vi "Global Mapper F.vi"(8 "picture in":picture, 11 "GIC Input":T1={"     Use ?\nOff       On"=[FALSE, TRUE, FALSE, TRUE], "Mode:"=FALSE, "WP Data"="", "Hokuyo Port"="COM7", "Prop  Port"="COM6", "Compass Port"="", "GPS Port"="", "Num of WPs"=0, "WP Lats and Longs"={"WP Lats"=[], "WP Longs"=[]}, "Obst Lats and Longs"={"Obst Lats"=[], "Obst Longs"=[]}, "Parameters"=[], "GPS Data"=[], "Compass"=0.0, "LMS Vector"=[], "Vision Vector"=[], "Direction Cmd"=0.0, "Speed Cmd"=0.0, "WP Vector"=[], "WP Number"=0, "Extra"=0, "SW Map"=[], "Path Cluster"={"Path x node"=[], "Path y node"=[]}, "Sim Course"=[]} {"Obst Lats and Longs"."Obst Longs" format="%#_8g"; "Obst Lats and Longs"."Obst Lats" format="%#_8g"}) -> (0 "picture out":picture)   [LabVIEW 2014]
panel:
  # "Global Mapper F"
  # "Inputs:"
  # "Output:"
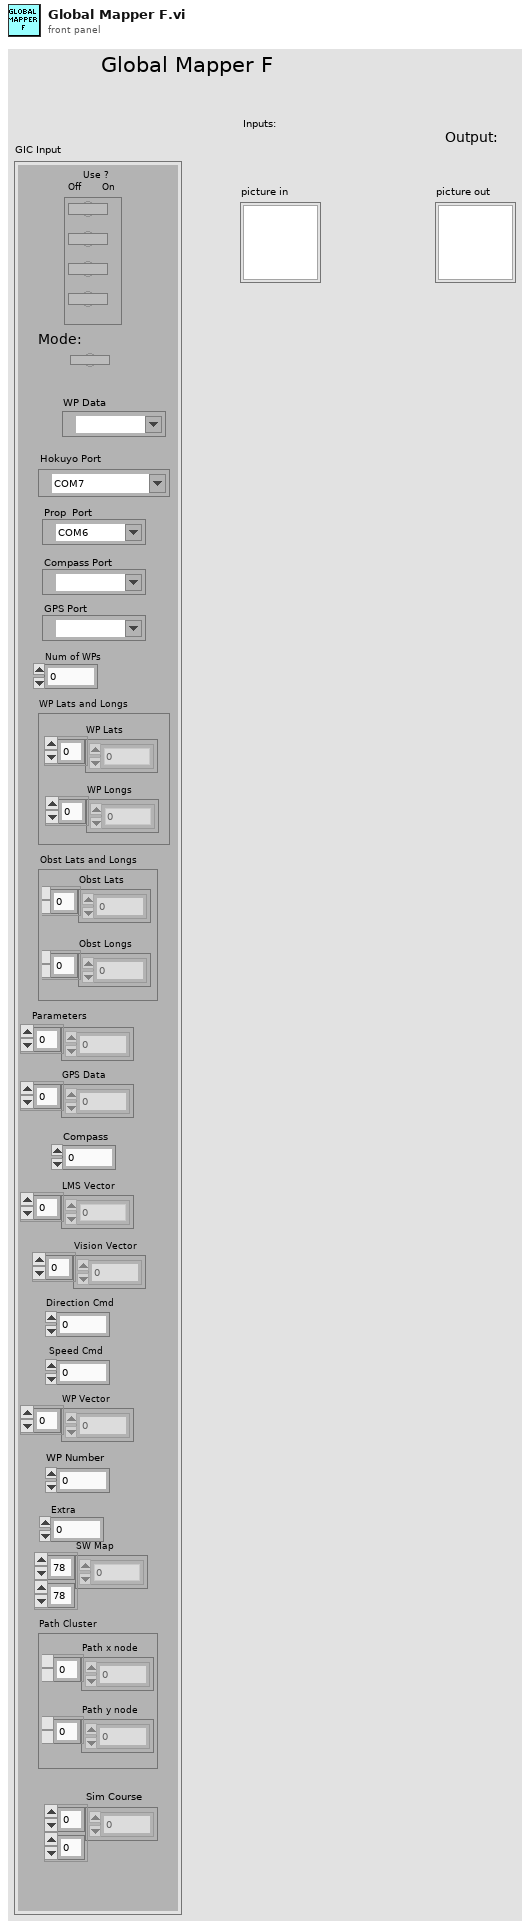
[diagram p1: front panel]
types:
  T1 = cluster{"     Use ?\nOff       On":bool[], "Mode:":bool, "WP Data":refnum<visa-resource-name>, "Hokuyo Port":refnum<visa-resource-name>, "Prop  Port":refnum<visa-resource-name>, "Compass Port":refnum<visa-resource-name>, "GPS Port":refnum<visa-resource-name>, "Num of WPs":i16, "WP Lats and Longs":cluster{"WP Lats":dbl[], "WP Longs":dbl[]}, "Obst Lats and Longs":cluster{"Obst Lats":dbl[], "Obst Longs":dbl[]}, "Parameters":dbl[], "GPS Data":dbl[], "Compass":dbl, "LMS Vector":dbl[], "Vision Vector":dbl[], "Direction Cmd":dbl, "Speed Cmd":dbl, "WP Vector":dbl[], "WP Number":i32, "Extra":i16, "SW Map":i32[][], "Path Cluster":cluster{"Path x node":dbl[], "Path y node":dbl[]}, "Sim Course":i8[][]}
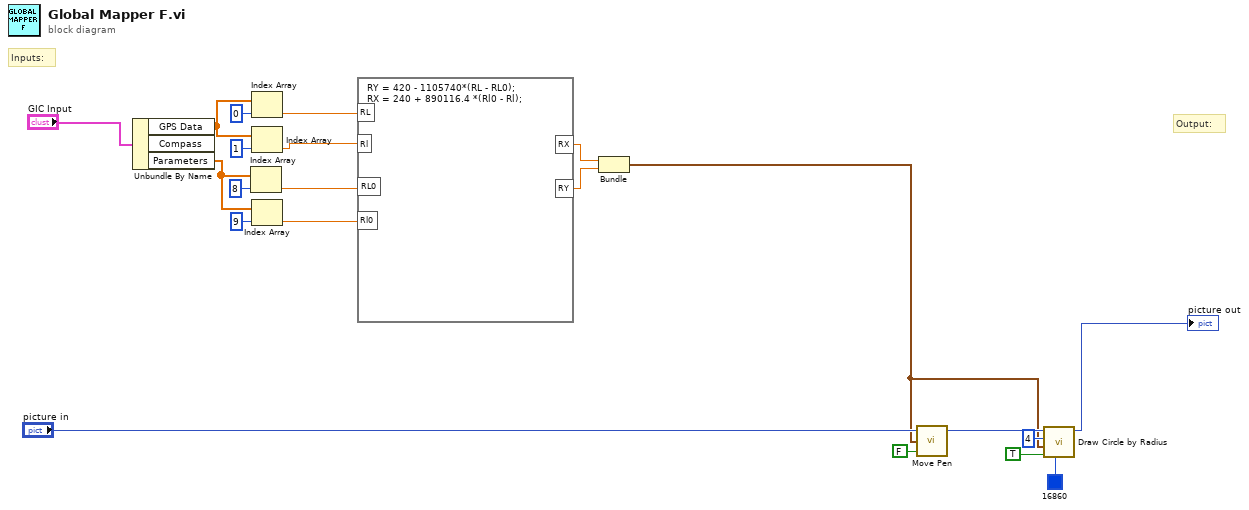
[diagram p0: block diagram]
diagram:
  # "Output:"
  # "Inputs:"
  n1 = Unbundle By Name("GIC Input") -> ("GPS Data"=w18:dbl[], "Parameters"=w13:dbl[])  [unwired: 1 out]
  n2 = Index Array(array=w13, index=8) -> (element=w15:dbl)
  n3 = Index Array(array=w18, index=0) -> (element=w20:dbl)
  n4 = Index Array(array=w18, index=1) -> (element=w16:dbl)
  n5 = Index Array(array=w13, index=9) -> (element=w11:dbl)
  n6 = formula code="RY = 420 - 1105740*(RL - RL0);\nRX = 240 + 890116.4 *(Rl0 - Rl);"("RL"=w20, "Rl"=w16, "RL0"=w15, "Rl0"=w11) -> ("RY"=w7:dbl, "RX"=w8:dbl)
  n7 = Bundle("RX"=w8, "RY"=w7) -> (w1:cluster{"RX":dbl, "RY":dbl})  [unwired: 1 in]
  n8 = call <vilib>:"Move Pen.vi"("absolute coordinates?(T)"=FALSE, "new position"=w1, "picture"="picture in") -> ("new picture"=w9:picture)  [unwired: 2 in]
  n9 = call <vilib>:"Draw Circle by Radius.vi"("color(black)"=u32 16860, "fill?(F)"=TRUE, "pixel center"=w1, "radius"=i16 4, "picture"=w9) -> ("new picture"=→"picture out":picture)  [unwired: 6 in]
